vi "Create Save Grid.vi"() -> ()   [LabVIEW 2013]
uses:
  Controls/Type of Neuron.ctl
  Cube/Grid.lvclass
panel:
  out "Progress":dbl
  out "error out":errorcluster
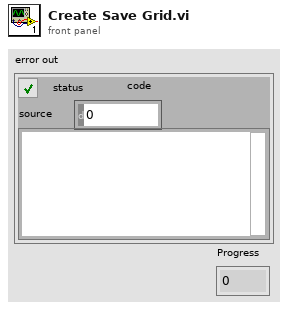
[diagram p1: front panel]
types:
  T1 = typedef "Type of Neuron.ctl" = enum16{"MF", "BA", "GO", "GC", "PC", "LU", "Glia (Dummy)"}
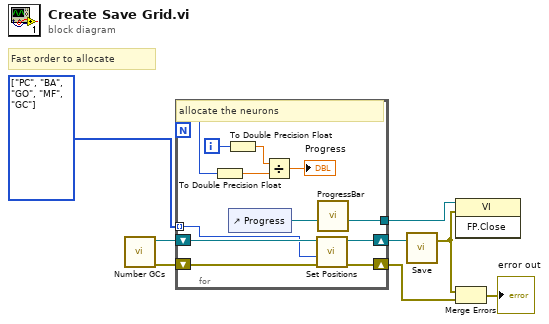
[diagram p0: block diagram]
diagram:
  w8 = T1[] [enum."PC", enum."BA", enum."GO", enum."MF", enum."GC"] items=["MF", "BA", "GO", "GC", "PC", "LU", "Glia (Dummy)"]
  # "Fast order to allocate"
  n1 = call "Number GCs.vi"() -> ("error out"=w3:errorcluster, "Cube out"=w6:refnum<class "Grid.lvclass">)  [unwired: 5 in, 2 out]
  n2 = for {
    N -> [w12]
    shift-right: [w19] -> w7
    shift-left: w6 -> [w20]
    tunnel: w8 -> [w16] mode=indexing
    shift-right: [w17] -> w5
    shift-left: w3 -> [w18]
    tunnel: [w9] -> w1
    i -> [w11]
    # "allocate the neurons"
    n3 = To Double Precision Float(number=w12) -> (double precision float=w15:dbl)
    n4 = To Double Precision Float(number=w11) -> (double precision float=w14:dbl)
    n5 = control-ref of="Progress"() -> (w10:refnum<vi>)
    n6 = Divide(x=w14, y=w15) -> (x/y=→"Progress":dbl)
    n7 = call "Set Positions.vi"("error in"=w18, "Type of Neuron"=w16, "Grid in"=w20) -> ("error out"=w17:errorcluster, "Grid out"=w19:refnum<class "Grid.lvclass">)  [unwired: 7 in]
    n8 = call "ProgressBar.vi"("Progress"=w10) -> ("This VI"=w9:refnum<vi>)  [unwired: 10 in]
  }
  n9 = call "Save.vi"("Grid in"=w7) -> ("error out"=w2:errorcluster)  [unwired: 1 in, 1 out]
  n10 = invoke class="VI" method="FP.Close"(reference=w1, error in=w2) -> ()  [unwired: 1 in, 3 out]
  n11 = Merge Errors(w2, w5) -> (→"error out":errorcluster)
